vi "Show all controls.vi"(6 "Variant in":variant, 7 "Shift Pressed?":bool, 8 "error in (no error)":errorcluster, 10 "QD Combo Box Ref":refnum<vi>, 11 "QD Launch VI Ref":refnum<vi>) -> (0 "error out":errorcluster, 4 "Variant out":variant)   [LabVIEW 2017]
doc: "Ensures that there are Error In and Error Out controls on the front panel, positioned above the origin and that they are attached to the connector pane terminals.\n\nDefault Shortcut - [V]"
uses:
  <vilib>/Utility/traverseref.llb/TRef TravTarget.ctl
  <vilib>/Utility/traverseref.llb/VI Scripting - Traverse.lvlib
panel:
  in  "Undo Name":string="Quick Drop Keyboard Shortcut"
  # "Do not change the connector pane of this VI.\n\nSee the block diagram for directions on how to use this template."
  # "Specify the name of the Undo transaction"
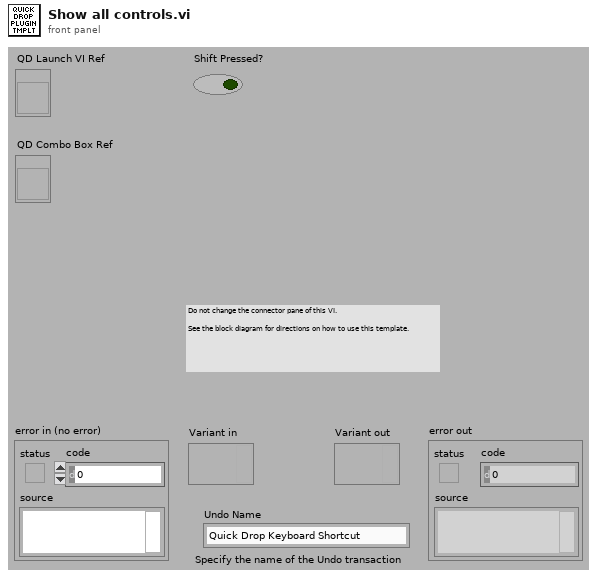
[diagram p1: front panel]
types:
  T1 = typedef "TRef TravTarget.ctl" = enum16{"FP", "BD", "Other"}
  T2 = enum8{"Enabled", "Disabled", "Disabled and Grayed Out"}
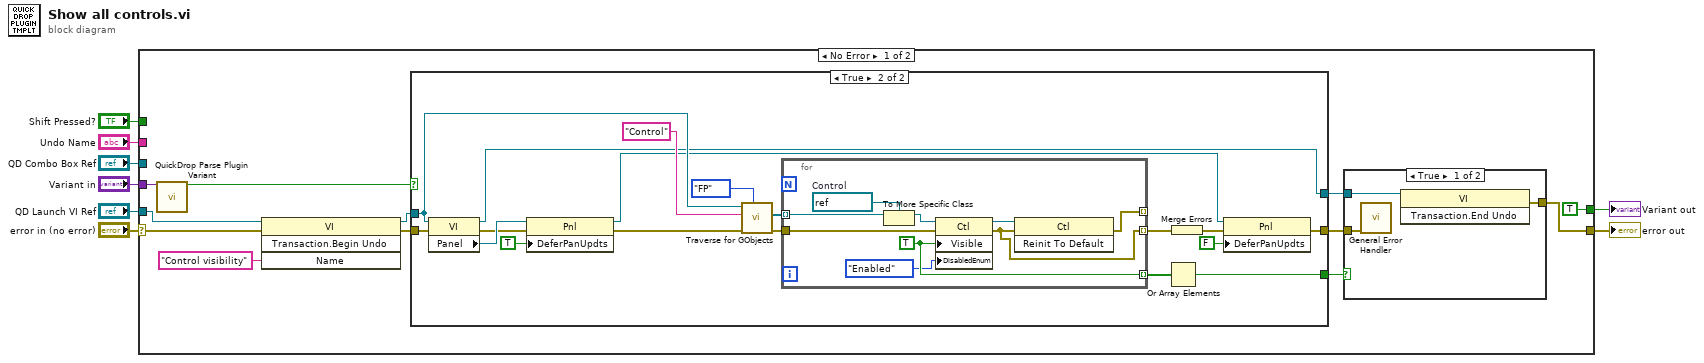
[diagram p0: block diagram]
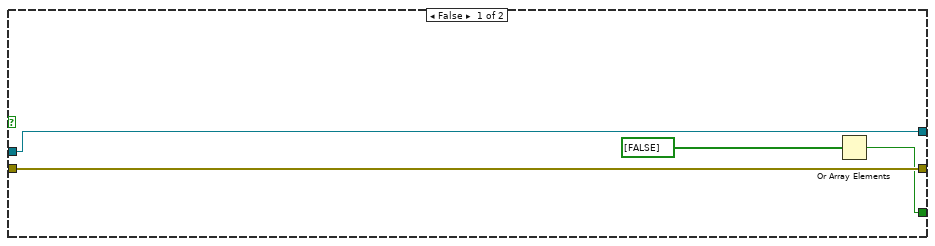
[diagram p2: hidden frame]
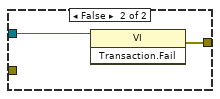
[diagram p3: hidden frame]
diagram:
  n1 = case shown="No Error" "error in (no error)" {
    selector: "error in (no error)" -> [w19 w57]
    tunnel: [w15 w57] -> w7
    tunnel: "QD Launch VI Ref" -> [w18 _]
    tunnel: "Shift Pressed?" -> [_ _]
    tunnel: "QD Combo Box Ref" -> [_ _]
    tunnel: "Variant in" -> [w20 _]
    tunnel: "Undo Name" -> [_ _]
    tunnel: [TRUE _] -> w1
    frame No Error {
      n2 = call <vilib>:"QuickDrop Parse Plugin Variant.vi"("QDKS Variant in"=w20) -> ("QD Launch VI Panel?"=w10:bool)  [unwired: 12 in, 2 out]
      n3 = invoke class="VI" method="Transaction.Begin Undo"(reference=w18, error in=w19, "Name"="Control visibility") -> (reference out=w13:refnum<vi>, error out=w16:errorcluster)  [unwired: 1 in, 2 out]
      n4 = case shown="True" w10 {
        tunnel: w16 -> [w24 w33]
        tunnel: [w24 w27] -> w14
        tunnel: w13 -> [w23 w41]
        tunnel: [w22 w42] -> w12
        tunnel: [w23 w36] -> w9
        frame False {
          n5 = Or Array Elements(Boolean array=bool[] [FALSE]) -> (logical OR=w22:bool)
        }
        frame True {
          n6 = property class="VI"(reference=w41, error in=w33) -> (reference out=w36:refnum<vi>, error out=w34:errorcluster, "Panel"=w35:refnum<vi>)
          n7 = property class="Pnl"(reference=w35, error in=w34, "DeferPanUpdts"=TRUE ("Defer Panel Updates")) -> (reference out=w26:refnum<vi>, error out=w32:errorcluster)
          n8 = call <vilib>:"Traverse for GObjects.vi"("Traverse Target"=TRef_TravTarget."FP", "error in (no error)"=w32, "Class Name"="Control", "VI Refnum"=w41) -> ("error out"=w31:errorcluster, "References"=w39:refnum<vi>[])  [unwired: 4 in, 2 out]
          n9 = for {
            tunnel: w39 -> [w51] mode=indexing
            tunnel: [w48] -> w37 mode=indexing
            tunnel: w31 -> [w46]
            tunnel: [w44] -> w30 mode=indexing
            tunnel: [w43] -> _ mode=indexing
            w48 = TRUE ("Visible")
            w49 = refnum<vi> refnum  # Control
            n10 = To More Specific Class(target class=w49, reference=w51) -> (specific class reference=w50:refnum<vi>)  [unwired: 1 in, 1 out]
            n11 = property class="Ctl"(reference=w50, error in=w46, "Visible"=w48, "DisabledEnum"=T2."Enabled" ("Disabled")) -> (reference out=w45:refnum<vi>, error out=w44:errorcluster)
            n12 = invoke class="Ctl" method="Reinit To Default"(reference=w45, error in=w44) -> (error out=w43:errorcluster)  [unwired: 1 in, 2 out]
          }
          n13 = Or Array Elements(Boolean array=w37) -> (logical OR=w42:bool)
          n14 = Merge Errors(w30) -> (w28:errorcluster)
          n15 = property class="Pnl"(reference=w26, error in=w28, "DeferPanUpdts"=FALSE ("Defer Panel Updates")) -> (error out=w27:errorcluster)  [unwired: 1 out]
        }
      }
      n16 = case shown="True" w12 {
        tunnel: w9 -> [w53 w55]
        tunnel: [w54 w56] -> w15
        tunnel: w14 -> [w52 _]
        frame True {
          n17 = call <vilib>:"General Error Handler.vi"("error in (no error)"=w52) -> ()  [unwired: 10 in, 5 out]
          n18 = invoke class="VI" method="Transaction.End Undo"(reference=w53) -> (error out=w54:errorcluster)  [unwired: 2 in, 2 out]
        }
        frame False {
          n19 = invoke class="VI" method="Transaction.Fail"(reference=w55) -> (error out=w56:errorcluster)  [unwired: 2 in, 2 out]
        }
      }
    }
    frame Error {
    }
  }
  "error out" <- w7
  "Variant out" <- w1
